vi "controls.vi"() -> ()   [LabVIEW 2019]
uses:
  ARCHIVE/Hydro4000/Old/LabVIEW 2019 Software 2022-02-22/Software/Graphics/Custom Valves/2 way energized.ctl
  ARCHIVE/Hydro4000/Old/LabVIEW 2019 Software 2022-02-22/Software/Graphics/Custom Valves/2 way_R.ctl
  ARCHIVE/Hydro4000/Old/LabVIEW 2019 Software 2022-02-22/Software/Graphics/Custom Valves/3 way energized.ctl
  ARCHIVE/Hydro4000/Old/LabVIEW 2019 Software 2022-02-22/Software/Graphics/Custom Valves/3 way valve.ctl
  ARCHIVE/Hydro4000/Old/LabVIEW 2019 Software 2022-02-22/Software/Graphics/Custom Valves/3Way_B_90degrees.ctl
  ARCHIVE/Hydro4000/Old/LabVIEW 2019 Software 2022-02-22/Software/Graphics/Custom Valves/3Way_BR.ctl
  ARCHIVE/Hydro4000/Old/LabVIEW 2019 Software 2022-02-22/Software/Graphics/Custom Valves/3Way_MV.ctl
  ARCHIVE/Hydro4000/Old/LabVIEW 2019 Software 2022-02-22/Software/Graphics/Custom Valves/3Way_UR_R.ctl
panel:
  in  "3 Way 6":T1
  in  "3 Way 5":T2
  in  "3 Way 4":T3
  in  "3 Way 3":T4
  in  "3 Way 2":T5
  in  "3 Way":T6
  in  "2 Way 2":T7
  in  "2 Way":T8
  out "Alarm Summary Data":T9
  in  "Read Parameters":T10={"Min priority"=0, "Max priority"=1000, "Show Acknowledged alarms?"=FALSE} {"Max priority" max=1000 step=1; "Min priority" max=1000 step=1}
  in  "alarm filter":T11={"start timestamp"=timestamp(0 s since 1904-01-01), "stop timestamp (now)"=timestamp(0 s since 1904-01-01), "project variable name"="", "process"="", "set user"="", "clear user"="", "ack user"="", "alarm area"="", "ack comment"="", "alarm description"="", "alarm setpoint"=0.0, "value at alarm"=0.0, "minimum priority"=-1, "maximum priority"=-1, "filter on..."={"start timestamp"=FALSE, "project variable name"=FALSE, "process"=FALSE, "set user"=FALSE, "clear user"=FALSE, "ack user"=FALSE, "alarm area"=FALSE, "ack comment"=FALSE, "alarm description"=FALSE, "alarm setpoint"=FALSE, "value at alarm"=FALSE, "minimum priority"=FALSE, "maximum results"=FALSE, "return newest entries first"=FALSE}, "show..."=0, "maximum results"=-1, "return newest entries first"=FALSE} {"show..." items=["alarms & events", "alarms", "events"]; "stop timestamp (now)" format="%<%X\n%x>T"; "start timestamp" format="%<%X\n%x>T"; "value at alarm" format="%.2f"; "alarm setpoint" format="%.2f"; "maximum priority" min=-1 max=1000 step=1; "minimum priority" min=-1 max=1000 step=1}
  out "alarm":T12 {"value" format="%.2f"; "setpoint" format="%.2f"; "clear time" format="%<%X\n%x>T"; "ack time" format="%<%X\n%x>T"; "set time" format="%<%X\n%x>T"}
  out "Tank 3":dbl(slide) scale=0.0..100.0
  out "Tank 2":dbl(slide) scale=0.0..100.0
  out "Hopper":dbl(slide) scale=0.0..100.0
  out "Tank":dbl(slide) scale=0.0..10.0
  out "Boolean 44":bool
  out "Boolean 43":bool
  out "Boolean 42":bool
  out "Boolean 41":bool
  out "Boolean 40":bool
  out "Boolean 39":bool
  out "Boolean 38":bool
  out "Boolean 37":bool
  out "Boolean 36":bool
  out "Boolean 35":bool
  out "Boolean 34":bool
  out "Boolean 33":bool
  out "Boolean 32":bool
  out "Boolean 31":bool
  out "Boolean 30":bool
  out "Boolean 29":bool
  out "Boolean 28":bool
  out "Boolean 27":bool
  out "Boolean 26":bool
  out "Boolean 25":bool
  out "Boolean 24":bool
  out "Boolean 23":bool
  out "Boolean 22":bool
  out "Boolean 21":bool
  out "Boolean 20":bool
  out "Boolean 19":bool
  out "Boolean 18":bool
  out "Boolean 17":bool
  out "Boolean 16":bool
  out "Boolean 15":bool
  out "Boolean 14":bool
  out "Boolean 13":bool
  out "Boolean 12":bool
  out "Boolean 11":bool
  out "Boolean 10":bool
  out "Boolean 9":bool
  out "Boolean 8":bool
  out "Boolean 7":bool
  out "Boolean 6":bool
  out "Boolean 5":bool
  out "Boolean 4":bool
  out "Boolean 3":bool
  out "Boolean 2":bool
  out "Boolean":bool
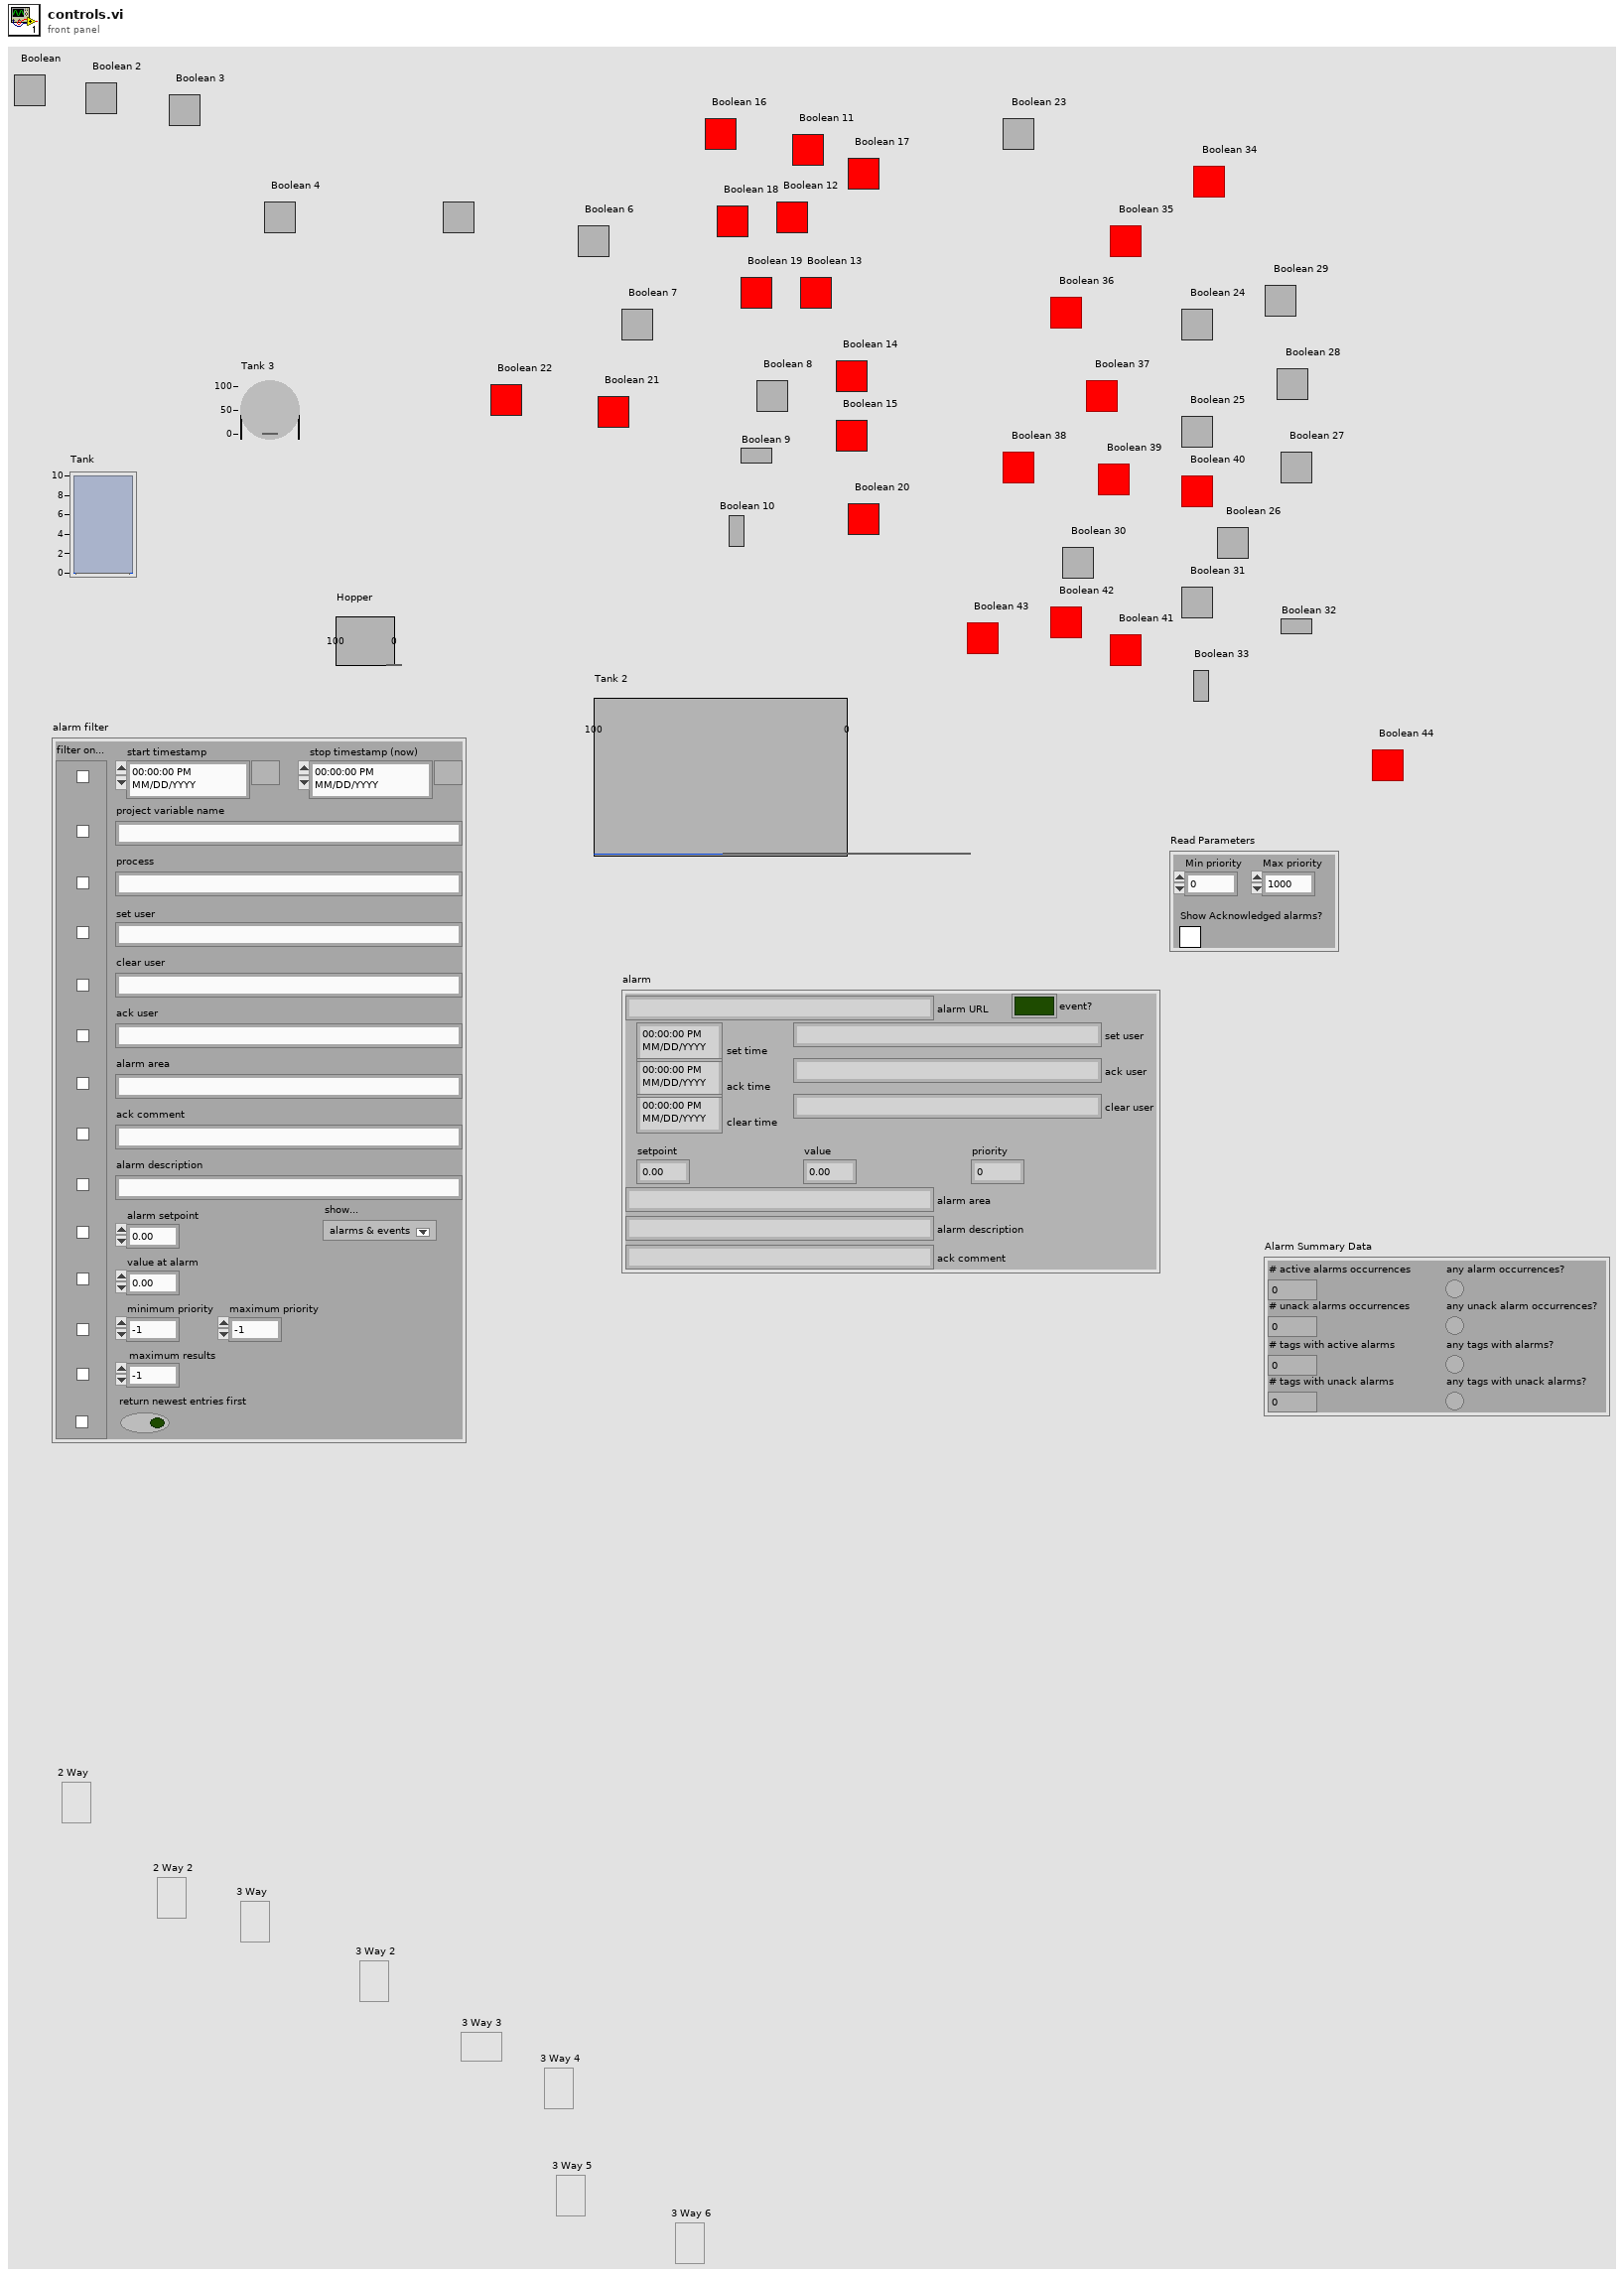
[diagram p1: front panel]
types:
  T1 = typedef "3Way_UR_R.ctl" = bool
  T2 = typedef "3Way_MV.ctl" = bool
  T3 = typedef "3Way_BR.ctl" = bool
  T4 = typedef "3Way_B_90degrees.ctl" = bool
  T5 = typedef "3 way valve.ctl" = bool
  T6 = typedef "3 way energized.ctl" = bool
  T7 = typedef "2 way_R.ctl" = bool
  T8 = typedef "2 way energized.ctl" = bool
  T9 = cluster{"# active alarms occurrences":i32, "any alarm occurrences?":bool, "# unack alarms occurrences":i32, "any unack alarm occurrences?":bool, "# tags with active alarms":i32, "any tags with alarms?":bool, "# tags with unack alarms":i32, "any tags with unack alarms?":bool}
  T10 = cluster{"Min priority":u32, "Max priority":u32, "Show Acknowledged alarms?":bool}
  T11 = cluster{"start timestamp":timestamp, "stop timestamp (now)":timestamp, "project variable name":string, "process":string, "set user":string, "clear user":string, "ack user":string, "alarm area":string, "ack comment":string, "alarm description":string, "alarm setpoint":dbl, "value at alarm":dbl, "minimum priority":i32, "maximum priority":i32, "filter on...":cluster{"start timestamp":bool, "project variable name":bool, "process":bool, "set user":bool, "clear user":bool, "ack user":bool, "alarm area":bool, "ack comment":bool, "alarm description":bool, "alarm setpoint":bool, "value at alarm":bool, "minimum priority":bool, "maximum results":bool, "return newest entries first":bool}, "show...":u16, "maximum results":i32, "return newest entries first":bool}
  T12 = cluster{"alarm URL":string, "set time":timestamp, "set user":string, "ack time":timestamp, "ack user":string, "clear time":timestamp, "clear user":string, "setpoint":dbl, "value":dbl, "priority":u32, "alarm area":string, "alarm description":string, "ack comment":string, "event?":bool, "Refnum":u64}
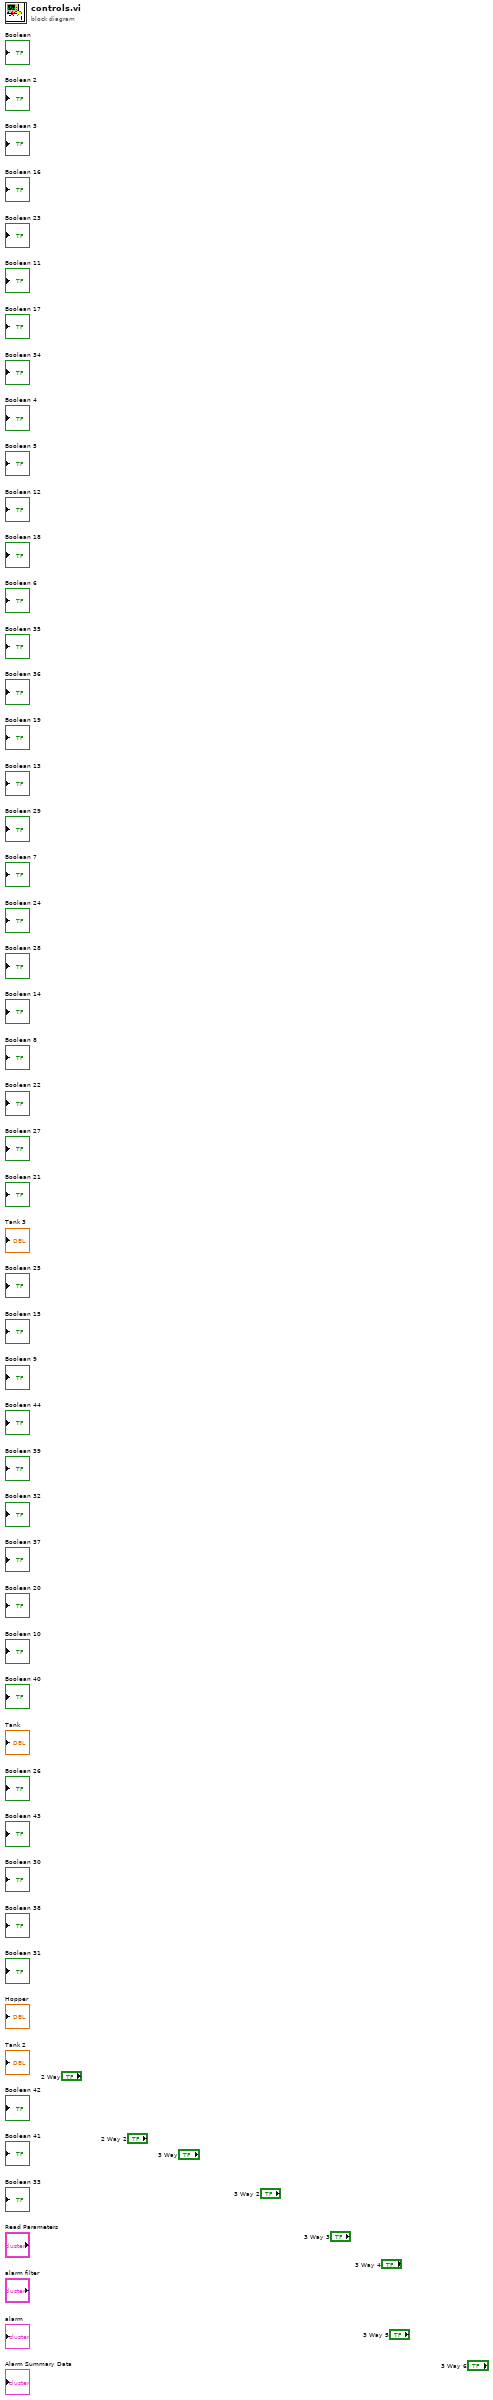
[diagram p0: block diagram]
diagram:
